vi "write acquisition config.vi"(8 "error in (no error)":errorcluster, 11 "Channel in":refnum<class "Channel.lvclass">) -> (0 "error out":errorcluster, 3 "Channel out":refnum<class "Channel.lvclass">)   [LabVIEW 2018, in "Channel.lvclass"]
uses:
  Channel.lvclass
  Channel.lvclass/Channel.ctl
  Sim_Ixon_Ultra/Sim_Ixon_Ultra.lvclass
  C:/Users/Denis/Desktop/S4ACS/S4ACS/Simulated_CCD_Camera/Simulated Camera.lvclass
  Simulated_CCD_Camera/Simulated Camera.lvclass
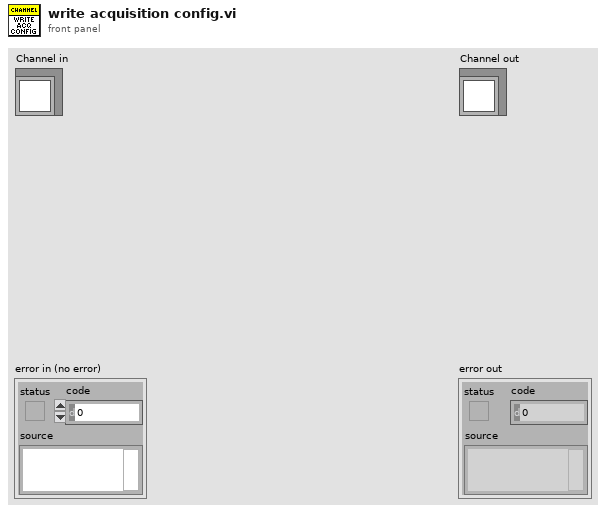
[diagram p1: front panel]
types:
  T1 = cluster{"EXPTIME":errorcluster, "#FRAMES":errorcluster}
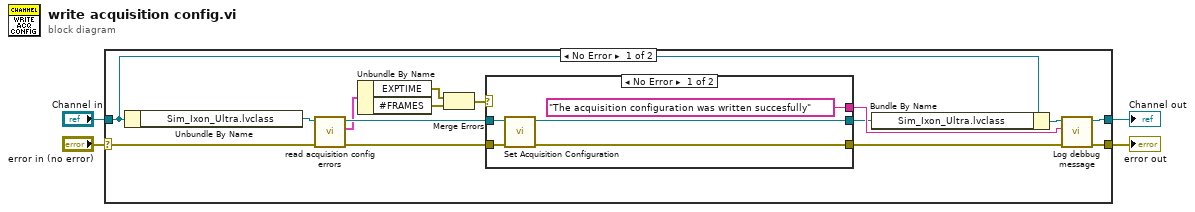
[diagram p0: block diagram]
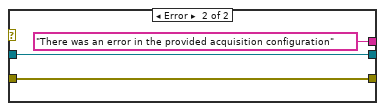
[diagram p2: hidden frame]
diagram:
  n1 = case shown="No Error" "error in (no error)" {
    selector: "error in (no error)" -> [w11 w29]
    tunnel: [w8 w29] -> w3
    tunnel: [w9 w28] -> w1
    tunnel: "Channel in" -> [w12 w28]
    frame No Error {
      n2 = Unbundle By Name(w12) -> ("Sim_Ixon_Ultra.lvclass"=w19:refnum<class "Sim_Ixon_Ultra.lvclass">)
      n3 = call "read acquisition config errors.vi"("error in (no error)"=w11, "Simulated Camera in"=w19) -> ("error out"=w17:errorcluster, "SET errors"=w16:T1, "Simulated Camera out"=w18:refnum<class "Sim_Ixon_Ultra.lvclass">)  [unwired: 7 in]
      n4 = Unbundle By Name(w16) -> ("EXPTIME"=w15:errorcluster, "#FRAMES"=w14:errorcluster)
      n5 = Merge Errors(w15, w14) -> (w13:errorcluster)
      n6 = case shown="No Error" w13 {
        tunnel: w18 -> [w23 w27]
        tunnel: w17 -> [w24 w26]
        tunnel: [w22 w26] -> w7
        tunnel: [w21 w27] -> w5
        tunnel: ["The acquisition configuration was written succesfully" ("String") "There was an error in the provided acquisition configuration" ("String")] -> w6
        frame No Error {
          n7 = call-dynamic "Set Acquisition Configuration.vi"("error in (no error)"=w24, "CCDCamera in"=w23) -> ("error out"=w22:errorcluster, "CCDCamera out"=w21:refnum<class "Sim_Ixon_Ultra.lvclass">)  [unwired: 8 in]
        }
        frame Error {
        }
      }
      n8 = Bundle By Name(cluster=w12, "Sim_Ixon_Ultra.lvclass"=w5) -> (w10:refnum<class "Channel.lvclass">)
      n9 = call "Log debbug message.vi"("error in (no error)"=w7, "String"=w6, "Channel in"=w10) -> ("error out"=w8:errorcluster, "Channel out"=w9:refnum<class "Channel.lvclass">)  [unwired: 7 in]
    }
    frame Error {
    }
  }
  "error out" <- w3
  "Channel out" <- w1
